vi "VictorPurpura.vi"(1 "template":i32[](array[numeric]), 2 "Test Object":i32[](array[numeric]), 3 "Cost":dbl) -> (0 "dissimilarity":dbl)   [LabVIEW 2018]
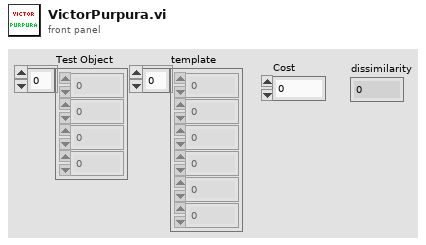
[diagram p1: front panel]
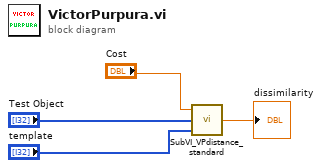
[diagram p0: block diagram]
diagram:
  n1 = call "SubVI_VPdistance_standard.vi"("Basis Object"="template", "Test Object"="Test Object", "Cost [1/ms]"="Cost") -> ("VP distance"=→"dissimilarity":dbl)
